vi "Unit Test - Test Add VI Reference Plugin.vi"() -> (0 "error out":errorcluster, 2 "Numeric 2":i32, 3 "Numeric":i32)   [LabVIEW 2017, in "testcase-csmhelper.lvclass"]
uses:
  testcase-csmhelper.lvclass
  src/user.lib/_NEVSTOP/Communicable State Machine(CSM)/_csmHelper/CSM-Helper.lvclass/CSM-Helper.ctl
  src/user.lib/_NEVSTOP/Communicable State Machine(CSM)/_csmHelper/Properties/Read Case Structure Ref.vi
  src/user.lib/_NEVSTOP/Communicable State Machine(CSM)/_csmHelper/API/Create From VI Reference.vi
  src/user.lib/_NEVSTOP/Communicable State Machine(CSM)/_csmHelper/API/Start Undo.vi
  src/user.lib/_NEVSTOP/Communicable State Machine(CSM)/_csmHelper/API/Remove State Frame.vi
  src/user.lib/_NEVSTOP/Communicable State Machine(CSM)/_csmHelper/API/Stop Undo.vi
  src/user.lib/_NEVSTOP/Communicable State Machine(CSM)/_csmHelper/API/Undo.vi
  src/user.lib/_NEVSTOP/Communicable State Machine(CSM)/_csmHelper/API/Destroy.vi
  src/user.lib/_NEVSTOP/Communicable State Machine(CSM)/_csmHelper/CSM-Helper.lvclass
  src/user.lib/_NEVSTOP/Communicable State Machine(CSM)/_csmHelper/Utility/_Support/CaseStructure.llb/csmHelper-CaseStructure.lvlib
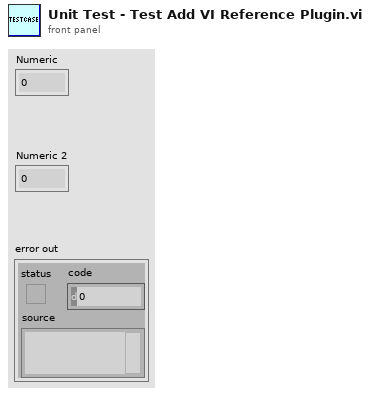
[diagram p1: front panel]
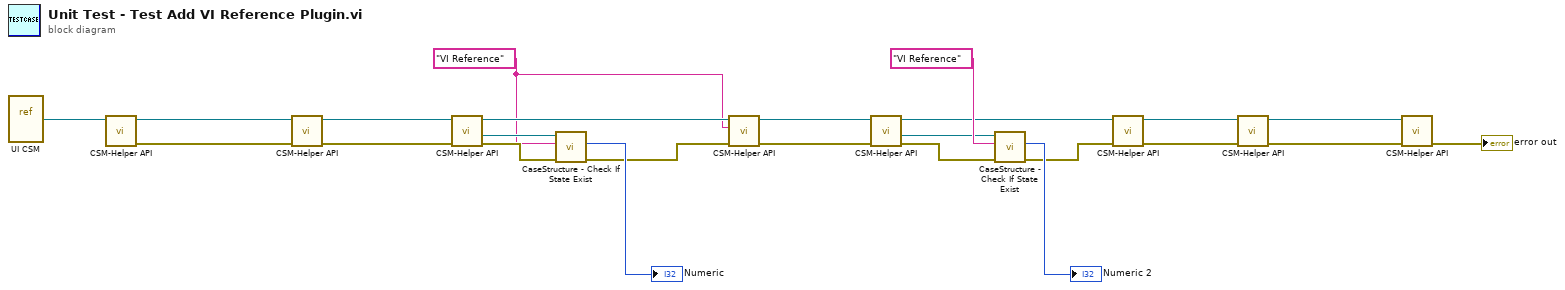
[diagram p0: block diagram]
diagram:
  w5 = "VI Reference" ("Group Name")
  n1 = vi-ref "UI CSM.vi"() -> (w24:refnum<vi>)
  n2 = call-poly "CSM-Helper API.vi"("VI"=w24) -> ("error out"=w19:errorcluster, "CSM-Helper.lvclass"=w18:refnum<class "CSM-Helper.lvclass">)  [unwired: 9 in]
  n3 = call-poly "CSM-Helper API.vi"("error in (no error)"=w19, "CSM-Helper in"=w18) -> ("error out"=w17:errorcluster, "CSM-Helper out"=w16:refnum<class "CSM-Helper.lvclass">)  [unwired: 8 in]
  n4 = call-poly "CSM-Helper API.vi"("error in (no error)"=w17, "CSM-Helper in"=w16) -> ("error out"=w22:errorcluster, "Case Structure"=w21:refnum<vi>, "CSM-Helper out"=w7:refnum<class "CSM-Helper.lvclass">)  [unwired: 7 in]
  n5 = call "CaseStructure - Check If State Exist.vi"("error in (no error)"=w22, "Group Name"=w5, "CaseStructure in"=w21) -> ("error out"=w6:errorcluster, "Numeric"=→"Numeric":i32)  [unwired: 6 in, 1 out]
  n6 = call-poly "CSM-Helper API.vi"("error in (no error)"=w6, "element"=w5, "CSM-Helper in"=w7) -> ("error out"=w4:errorcluster, "CSM-Helper out"=w3:refnum<class "CSM-Helper.lvclass">)  [unwired: 7 in]
  n7 = call-poly "CSM-Helper API.vi"("error in (no error)"=w4, "CSM-Helper in"=w3) -> ("error out"=w8:errorcluster, "Case Structure"=w9:refnum<vi>, "CSM-Helper out"=w2:refnum<class "CSM-Helper.lvclass">)  [unwired: 7 in]
  n8 = call "CaseStructure - Check If State Exist.vi"("error in (no error)"=w8, "Group Name"="VI Reference", "CaseStructure in"=w9) -> ("error out"=w1:errorcluster, "Numeric"=→"Numeric 2":i32)  [unwired: 6 in, 1 out]
  n9 = call-poly "CSM-Helper API.vi"("error in (no error)"=w1, "CSM-Helper in"=w2) -> ("error out"=w15:errorcluster, "CSM-Helper out"=w14:refnum<class "CSM-Helper.lvclass">)  [unwired: 8 in]
  n10 = call-poly "CSM-Helper API.vi"("error in (no error)"=w15, "CSM-Helper in"=w14) -> ("error out"=w13:errorcluster, "CSM-Helper out"=w12:refnum<class "CSM-Helper.lvclass">)  [unwired: 8 in]
  n11 = call-poly "CSM-Helper API.vi"("error in (no error)"=w13, "CSM-Helper in"=w12) -> ("error out"=→"error out":errorcluster)  [unwired: 8 in, 1 out]
